vi "Preview.vi"(8 "error in (no error)":errorcluster, 11 "BroadcastRegistry In":T1) -> (0 "error out":errorcluster, 2 "Registry":variant, 3 "BroadcastRegistry Out":T1)   [LabVIEW 2017, in "Communicable State Machine.lvlib"]
doc: "### Preview.vi\n\n-- <b>Controls</b> --\n- <b>BroadcastRegistry in</b>:\n\n-- <b>Indicators</b> --\n- <b>Registry</b>:\n- <b>BroadcastRegistry out</b>:"
uses:
  Communicable State Machine.lvlib
  BroadcastRegistry.ctl
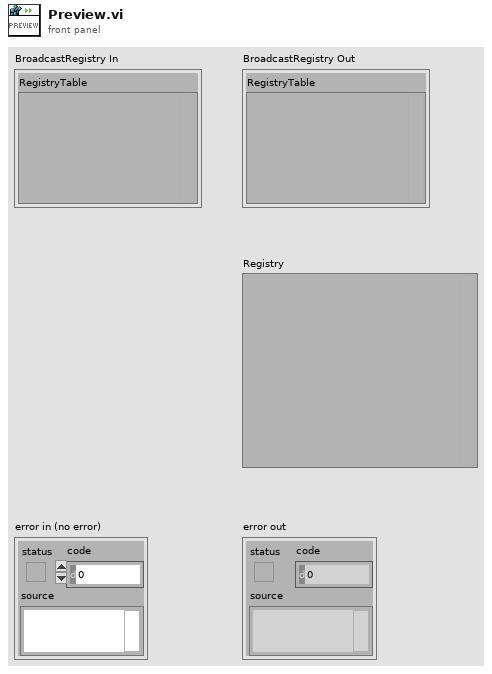
[diagram p1: front panel]
types:
  T1 = typedef "Communicable State Machine.lvlib/BroadcastRegistry.ctl" = cluster{"RegistryTable":variant}
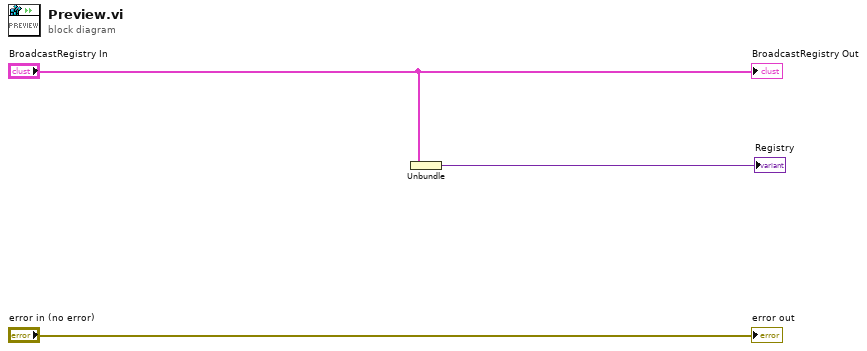
[diagram p0: block diagram]
diagram:
  n1 = Unbundle("BroadcastRegistry In") -> ("RegistryTable"=→"Registry":variant)
  "error out" <- "error in (no error)"
  "BroadcastRegistry Out" <- "BroadcastRegistry In"
